vi "HP-getBytesAtPort.vi"(8 "error in (no error)":errorcluster, 11 "HP-S-Serial in":refnum<class "HP-S-Serial.lvclass">) -> (0 "error out":errorcluster, 2 "Serial Settings:Number of Bytes at Serial Port":u32, 3 "HP-S-Serial out":refnum<class "HP-S-Serial.lvclass">)   [LabVIEW 2020, in "HP-S-Serial.lvclass"]
uses:
  HP-S-Serial.lvclass
  HP-S-Serial.lvclass/HP-S-Serial.ctl
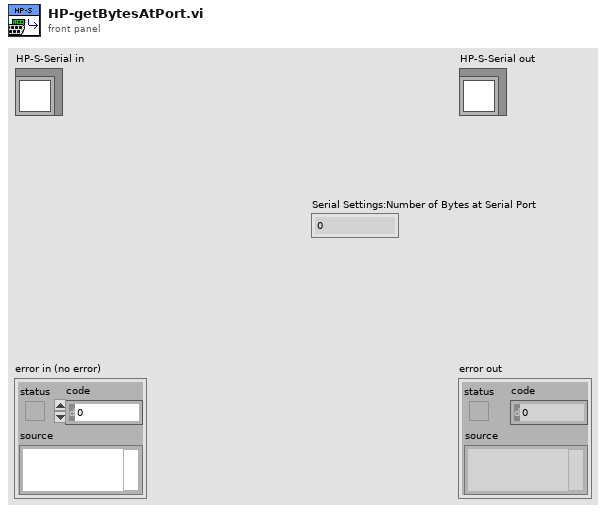
[diagram p1: front panel]
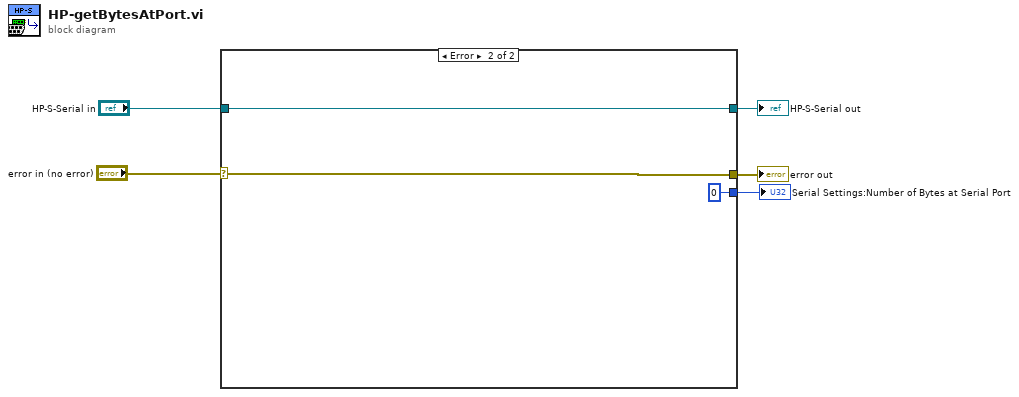
[diagram p0: block diagram]
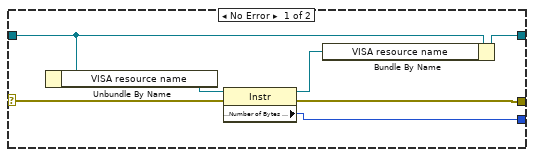
[diagram p2: hidden frame]
diagram:
  n1 = case shown="Error" "error in (no error)" {
    selector: "error in (no error)" -> [w9 w15]
    tunnel: [w7 w15] -> w4
    tunnel: [w10 w14] -> w2
    tunnel: "HP-S-Serial in" -> [w12 w14]
    tunnel: [w6 u32 0 ("Bytes at Port")] -> w1
    frame No Error {
      n2 = Unbundle By Name(w12) -> ("VISA resource name"=w11:refnum<visa-resource-name>)
      n3 = property class="Instr"(reference=w11, error in=w9) -> (reference out=w8:refnum<visa-resource-name>, error out=w7:errorcluster, "Serial Settings:Number of Bytes at Serial Port"=w6:u32)
      n4 = Bundle By Name(cluster=w12, "VISA resource name"=w8) -> (w10:refnum<class "HP-S-Serial.lvclass">)
    }
    frame Error {
    }
  }
  "error out" <- w4
  "HP-S-Serial out" <- w2
  "Serial Settings:Number of Bytes at Serial Port" <- w1
